vi "DMC CLI VI Analyzer Command Line Example.vi"() -> ()   [LabVIEW 2023]
panel:
  in  "Per VI Threshold?":bool
  out "standard error":string
  in  "Working Directory":path=path ""
  out "error out":errorcluster
  out "return code":i32
  out "standard output":string
  in  "Run VI Analyzer?":bool
  out "CMD String":string
  in  "RSL Report?":bool
  in  "HTML Report?":bool=TRUE
  in  "Thresholds":cluster{"High":dbl, "Normal":dbl, "Low":dbl}={"High"=100.0, "Normal"=100.0, "Low"=100.0}
  in  "Excluded Folders":string[](array[string])
  in  "Included Folders":string[](array[string])
  in  "Report Directory":path
  in  "Viancfg File Path":path
  in  "LabVIEW Year":string="2023"
  in  "Timeout (ms)":i32=240000
  # "g-cli --lv-ver [LV_Year] --arch 64 --timeout [ms Timeout] \"DMC CLI VI Analyzer\" -- [arguments]\n\n-------optional arguments-------\n-viancfg <absolute or relative to working directory relative path to viancfg file. defaults to Default.viancfg included with app>\n-reportdir <absolute or relative to working directory relative path to report output directory. Defaults to workingdir/Reports>\n-included <comma seperated string of all folders within working directory to include. Recursive search. Defaults to settings within viancfg>\n-excluded <comma seperated string of all folders within working directory to exclude. Defaults to none>\n-high <High Threshold, default 100>\n-normal <Normal Threshold, default 100>\n-low <Low Threshold, default 100>\n-pervi <Flag to run thresholds against each VI instead of catagories>\n-html <Flag to generate html report>\n-rsl <Flag to generate rsl report>\n-help <Returns this help information>"
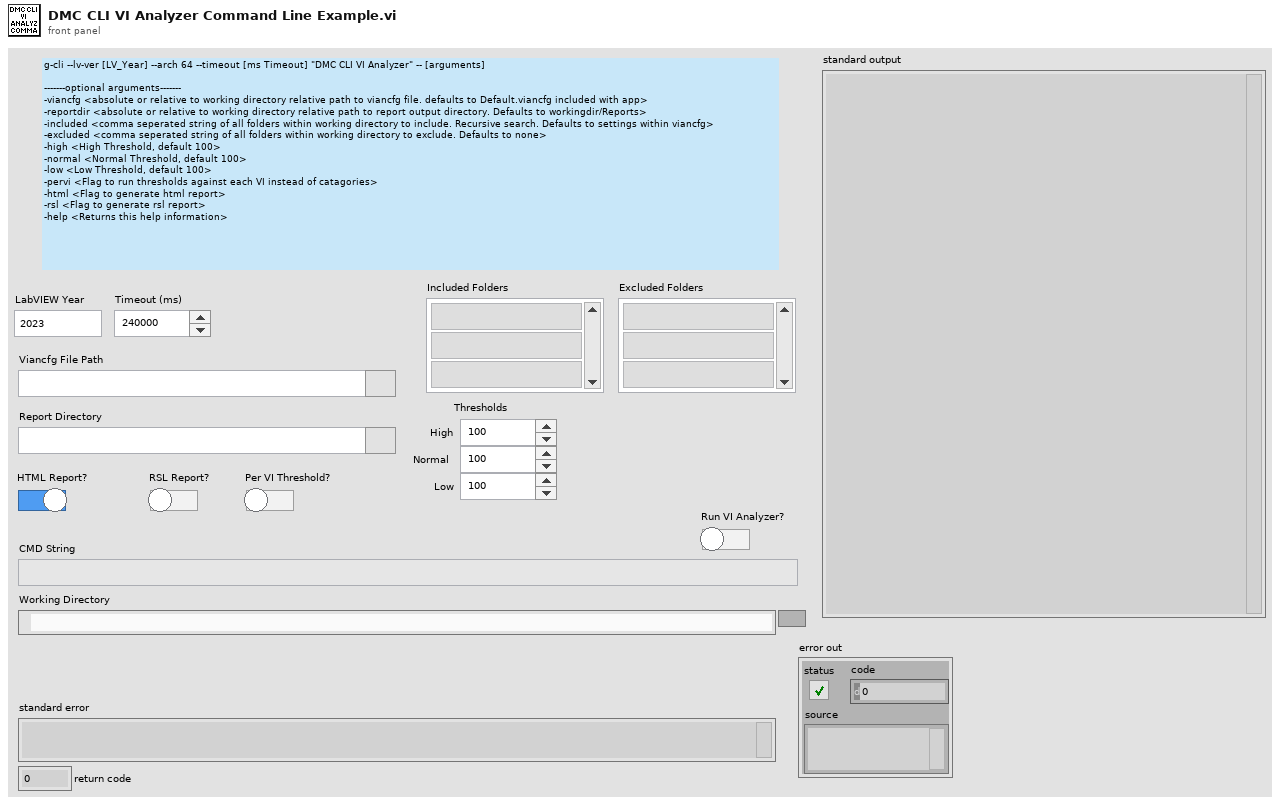
[diagram p1: front panel]
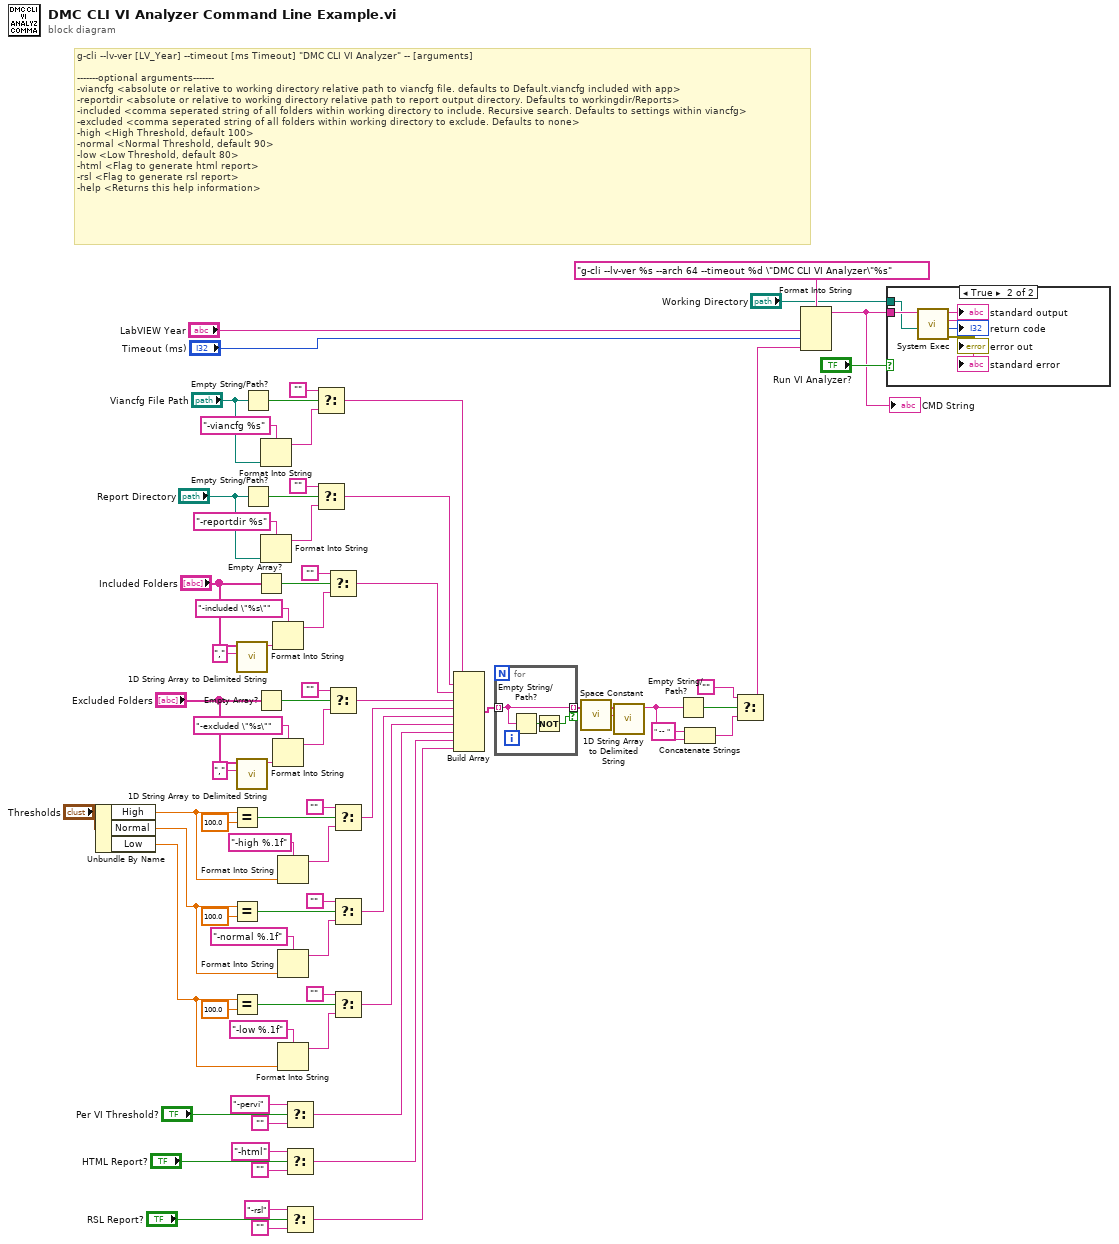
[diagram p0: block diagram]
diagram:
  # "g-cli --lv-ver [LV_Year] --timeout [ms Timeout] \"DMC CLI VI Analyzer\" -- [arguments]\n\n-------optional arguments-------\n-viancfg <absolute or relative to working directory relative path to viancfg file. defaults to Default.viancfg included with app>\n-reportdir <absolute or relative to working directory relative path to report output directory. Defaults to workingdir/Reports>\n-included <comma seperated string of all folders within working directory to include. Recursive search. Defaults to settings within viancfg>\n-excluded <comma seperated string of all folders within working directory to exclude. Defaults to none>\n-high <High Threshold, default 100>\n-normal <Normal Threshold, default 90>\n-low <Low Threshold, default 80>\n-html <Flag to generate html report>\n-rsl <Flag to generate rsl report>\n-help <Returns this help information>"
  n1 = Unbundle By Name("Thresholds") -> ("High"=w44:dbl, "Normal"=w33:dbl, "Low"=w32:dbl)
  n2 = Equal?(x=w44, y=100.0) -> (x = y?=w45:bool)
  n3 = Equal?(x=w33, y=100.0) -> (x = y?=w43:bool)
  n4 = Equal?(x=w32, y=100.0) -> (x = y?=w34:bool)
  n5 = call <vilib>:"1D String Array to Delimited String.vi"("delimiter"=",", "string array"="Included Folders") -> ("delimited string"=w59:string)  [unwired: 9 in]
  n6 = call <vilib>:"1D String Array to Delimited String.vi"("delimiter"=",", "string array"="Excluded Folders") -> ("delimited string"=w56:string)  [unwired: 9 in]
  n7 = Empty String/Path?(string/path="Viancfg File Path") -> (empty?=w74:bool)
  n8 = Empty String/Path?(string/path="Report Directory") -> (empty?=w66:bool)
  n9 = Empty Array?(array="Included Folders") -> (empty?=w58:bool)
  n10 = Empty Array?(array="Excluded Folders") -> (empty?=w57:bool)
  n11 = Format Into String(format string="-viancfg %s", "Viancfg File Path") -> (resulting string=w70:string)  [unwired: 2 in, 1 out]
  n12 = Format Into String(format string="-reportdir %s", "Report Directory") -> (resulting string=w69:string)  [unwired: 2 in, 1 out]
  n13 = Format Into String(format string="-included \"%s\"", w59) -> (resulting string=w64:string)  [unwired: 2 in, 1 out]
  n14 = Format Into String(format string="-excluded \"%s\"", w56) -> (resulting string=w52:string)  [unwired: 2 in, 1 out]
  n15 = Format Into String(format string="-high %.1f", w44) -> (resulting string=w46:string)  [unwired: 2 in, 1 out]
  n16 = Format Into String(format string="-normal %.1f", w33) -> (resulting string=w42:string)  [unwired: 2 in, 1 out]
  n17 = Format Into String(format string="-low %.1f", w32) -> (resulting string=w35:string)  [unwired: 2 in, 1 out]
  n18 = Select(t="-pervi", s="Per VI Threshold?", f="") -> (s? t:f=w1:string)
  n19 = Select(t="-html", s="HTML Report?", f="") -> (s? t:f=w18:string)
  n20 = Select(t="-rsl", s="RSL Report?", f="") -> (s? t:f=w17:string)
  n21 = Select(t="", s=w74, f=w70) -> (s? t:f=w25:string)
  n22 = Select(t="", s=w66, f=w69) -> (s? t:f=w24:string)
  n23 = Select(t="", s=w58, f=w64) -> (s? t:f=w23:string)
  n24 = Select(t="", s=w57, f=w52) -> (s? t:f=w22:string)
  n25 = Select(t="", s=w45, f=w46) -> (s? t:f=w21:string)
  n26 = Select(t="", s=w43, f=w42) -> (s? t:f=w20:string)
  n27 = Select(t="", s=w34, f=w35) -> (s? t:f=w19:string)
  n28 = Build Array(w25, w24, w23, w22, w21, w20, w19, w1, w18, w17) -> (w7:string[])
  n29 = for {
    tunnel: w7 -> [w80] mode=indexing
    tunnel: [w80] -> w6 mode=indexing if=w78
    n30 = Empty String/Path?(string/path=w80) -> (empty?=w79:bool)
    n31 = Not(x=w79) -> (.not. x?=w78:bool)
  }
  n32 = call <vilib>:"Space Constant.vi"() -> ("String"=w16:string)
  n33 = call <vilib>:"1D String Array to Delimited String.vi"("delimiter"=w16, "string array"=w6) -> ("delimited string"=w15:string)  [unwired: 9 in]
  n34 = Empty String/Path?(string/path=w15) -> (empty?=w13:bool)
  n35 = Concatenate Strings(" -- " ("string"), w15) -> (w11:string)
  n36 = Select(t="", s=w13, f=w11) -> (s? t:f=w10:string)
  n37 = Format Into String(format string="g-cli --lv-ver %s --arch 64 --timeout %d \"DMC CLI VI Analyzer\"%s", "LabVIEW Year", "Timeout (ms)", w10) -> (resulting string=w8:string)  [unwired: 2 in, 1 out]
  "CMD String" <- w8
  n38 = case shown="True" "Run VI Analyzer?" {
    tunnel: w8 -> [_ w86]
    tunnel: "Working Directory" -> [_ w82]
    frame False {
    }
    frame True {
      n39 = call <vilib>:"System Exec.vi"("working directory"=w82, "command line"=w86) -> ("error out"=→"error out":errorcluster, "return code"=→"return code":i32, "standard error"=→"standard error":string, "standard output"=→"standard output":string)  [unwired: 6 in]
    }
  }
